vi "Test1.vi"(10 "B":i32, 11 "A":i32) -> (2 "D":i32, 3 "C":i32)   [LabVIEW 2017]
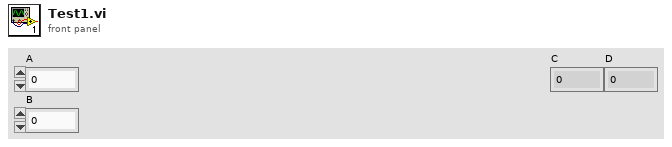
[diagram p1: front panel]
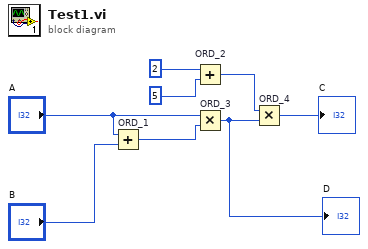
[diagram p0: block diagram]
diagram:
  n1 = Add "ORD_1"(x="A", y="B") -> (x+y=w7:i32)
  n2 = Add "ORD_2"(x=2, y=5) -> (x+y=w4:i32)
  n3 = Multiply "ORD_3"(x="A", y=w7) -> (x*y=w1:i32)
  "D" <- w1
  n4 = Multiply "ORD_4"(x=w4, y=w1) -> (x*y=→"C":i32)
